vi "8t008.vi"(1 "Input":string) -> (0 "Output":string)   [LabVIEW 2013]
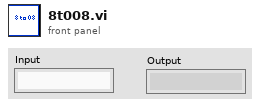
[diagram p1: front panel]
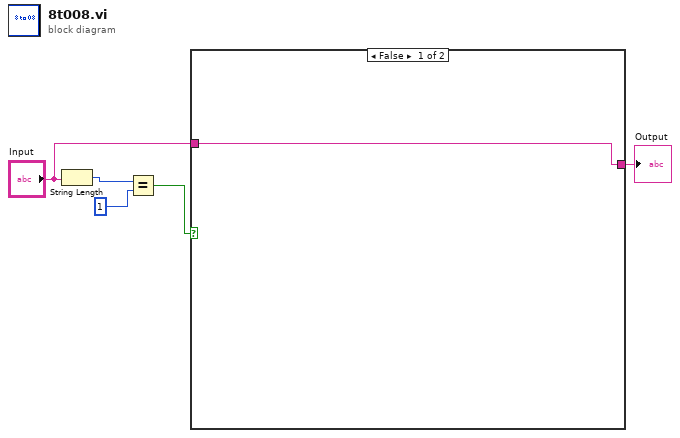
[diagram p0: block diagram]
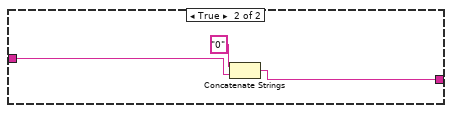
[diagram p2: hidden frame]
diagram:
  n1 = String Length(string="Input") -> (length=w5:i32)
  n2 = Equal?(x=w5, y=1) -> (x = y?=w2:bool)
  n3 = case shown="False" w2 {
    tunnel: "Input" -> [w6 w9]
    tunnel: [w6 w7] -> w1
    frame False {
    }
    frame True {
      n4 = Concatenate Strings("0" ("string"), w9) -> (w7:string)
    }
  }
  "Output" <- w1
